vi "get DVRs Refs.vi"() -> (2 "Controls":refnum<vi>[](array[refnum]))   [LabVIEW 2018]
uses:
  <vilib>/Utility/traverseref.llb/VI Scripting - Traverse.lvlib
  <vilib>/Utility/traverseref.llb/TRef TravTarget.ctl
panel:
  out "error out":errorcluster
  in  "error in (no error)":errorcluster
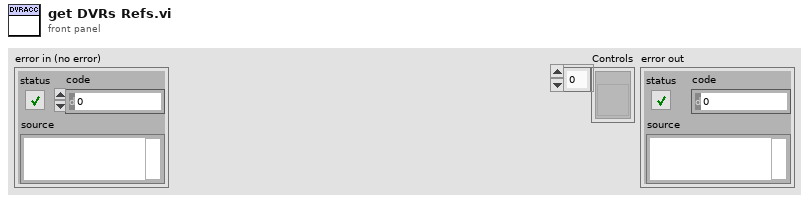
[diagram p1: front panel]
types:
  T1 = typedef "TRef TravTarget.ctl" = enum16{"FP", "BD", "Other"}
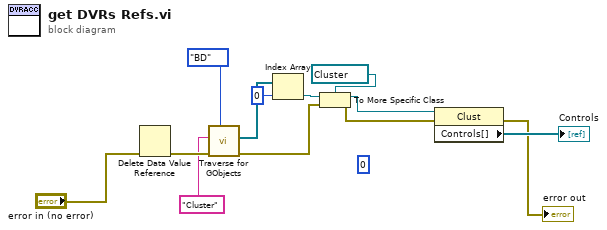
[diagram p0: block diagram]
diagram:
  (unwired) 0
  n1 = Delete Data Value Reference(error in="error in (no error)") -> (error out=w3:errorcluster)  [unwired: 1 in, 1 out]
  n2 = call <vilib>:"Traverse for GObjects.vi"("Traverse Target"=TRef_TravTarget."BD", "error in (no error)"=w3, "Class Name"="Cluster") -> ("error out"=w5:errorcluster, "References"=w10:refnum<vi>[])  [unwired: 5 in, 2 out]
  n3 = Index Array(array=w10, index=0) -> (element=w8:refnum<vi>)
  n4 = To More Specific Class(target class=refnum<vi> refnum ("Numeric"), reference=w8, error in=w5) -> (specific class reference=w6:refnum<vi>, error out=w4:errorcluster)
  n5 = property class="Clust"(reference=w6, error in=w4) -> (error out=→"error out":errorcluster, "Controls[]"=→"Controls":refnum<vi>[])  [unwired: 1 out]
